vi "SetPause.vi"(8 "error in (no error)":errorcluster, 11 "CameraSession in":refnum<class "CS250-CameraHardwareClass.lvclass">) -> (0 "error out":errorcluster, 3 "CameraSession out":refnum<class "CS250-CameraHardwareClass.lvclass">)   [LabVIEW 2013, in "CS250-CameraHardwareClass.lvclass"]
uses:
  CS250-CameraHardwareClass.lvclass
  CS250-CameraHardwareClass.lvclass/CS250-CameraHardwareClass.ctl
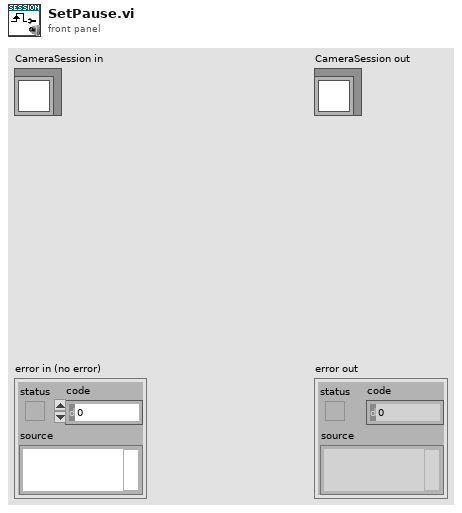
[diagram p1: front panel]
types:
  T1 = typedef "TriggerMode_TypDef.ctl" = enum16{"Timed", "Strobed", "Bulb", "Trigger first", "Flash", "Variable Timed"}
  T2 = typedef "OnOffTypeDef.ctl" = enum16{"off", "on"}
  T3 = typedef "CamCluster.ctl" = cluster{"hcam out":i16, "TempImage":T4, "Pointer":u32, "exp_bytes out":u32, "rgn_array":cluster{"s1":u16, "s2":u16, "sbin":u16, "p1":u16, "p2":u16, "pbin":u16}, "CameraName":string}
  T4 = typedef "IMAQ Image.ctl" = refnum<image>
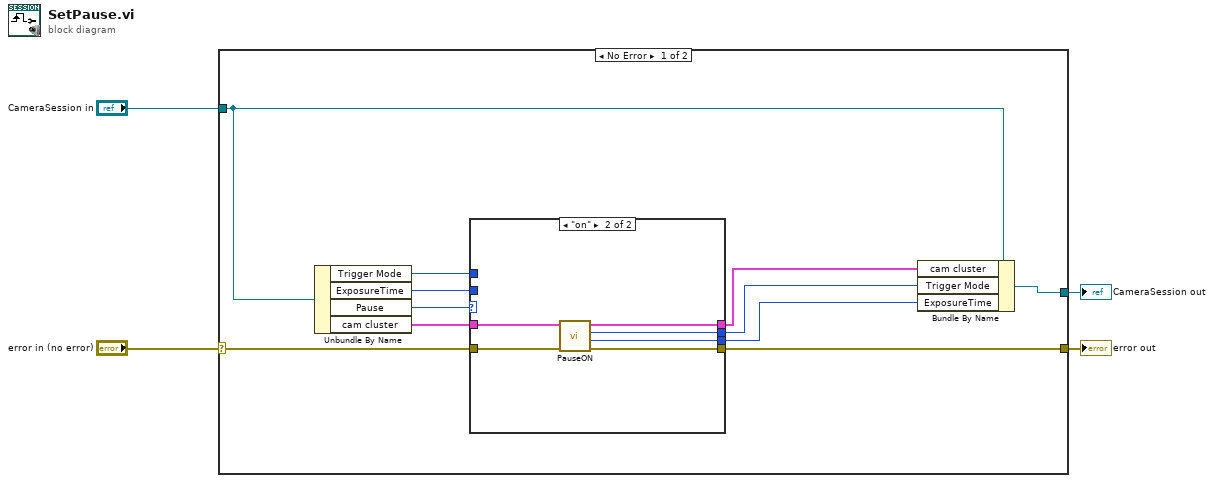
[diagram p0: block diagram]
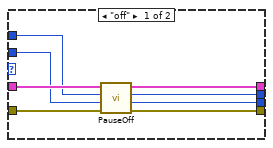
[diagram p2: hidden frame]
diagram:
  n1 = case shown="No Error" "error in (no error)" {
    selector: "error in (no error)" -> [w13 w31]
    tunnel: [w11 w31] -> w3
    tunnel: [w15 w30] -> w1
    tunnel: "CameraSession in" -> [w14 w30]
    frame No Error {
      n2 = Unbundle By Name(w14) -> ("Trigger Mode"=w5:T1, "ExposureTime"=w6:u32, "Pause"=w9:T2, "cam cluster"=w12:T3)
      n3 = case shown="\"on\"" w9 {
        tunnel: w13 -> [w23 w29]
        tunnel: [w21 w28] -> w11
        tunnel: w12 -> [w22 w27]
        tunnel: [w20 w26] -> w10
        tunnel: [w17 w25] -> w8
        tunnel: [w16 w24] -> w7
        tunnel: w6 -> [w18 _]
        tunnel: w5 -> [w19 _]
        frame "off" {
          n4 = call "PauseOff.vi"("error in (no error)"=w23, "exposure(ms)"=w18, "triggerModeIn"=w19, "cam cluster out in"=w22) -> ("error out"=w21:errorcluster, "exposure(ms) Out"=w16:u32, "triggerMode Out"=w17:T1, "cam cluster out"=w20:T3)  [unwired: 4 in]
        }
        frame "on" {
          n5 = call "PauseON.vi"("error in (no error)"=w29, "cam cluster out in"=w27) -> ("error out"=w28:errorcluster, "exposure (ms)"=w24:u32, "trigger mode"=w25:T1, "cam cluster out"=w26:T3)  [unwired: 6 in]
        }
      }
      n6 = Bundle By Name(cluster=w14, "cam cluster"=w10, "Trigger Mode"=w8, "ExposureTime"=w7) -> (w15:refnum<class "CS250-CameraHardwareClass.lvclass">)
    }
    frame Error {
    }
  }
  "error out" <- w3
  "CameraSession out" <- w1
